vi "Set Travel Speed to Min or Max.vi"(8 "error in (no error)":errorcluster, 10 "Travel Speed":T1=enum."Minimum", 11 "ESM303 in":refnum<class "ESM303.lvclass">) -> (0 "error out":errorcluster, 3 "ESM303 out":refnum<class "ESM303.lvclass">)   [LabVIEW 2018, in "ESM303.lvlib" / "ESM303.lvclass"]
uses:
  ESM303.lvclass
  builds/Force Test Stand/Force Test Stand/Force Test Stand.lvlibp/Custom Controls/Travel Speed.ctl
  builds/Force Test Stand/Force Test Stand/Force Test Stand.lvlibp/Force Test Stand.lvclass
  C:/Projects/LabVIEW/In-Progress/Jose Rivero-Diaz/builds/Force Test Stand/Force Test Stand/Force Test Stand.lvlibp/Force Test Stand.lvclass
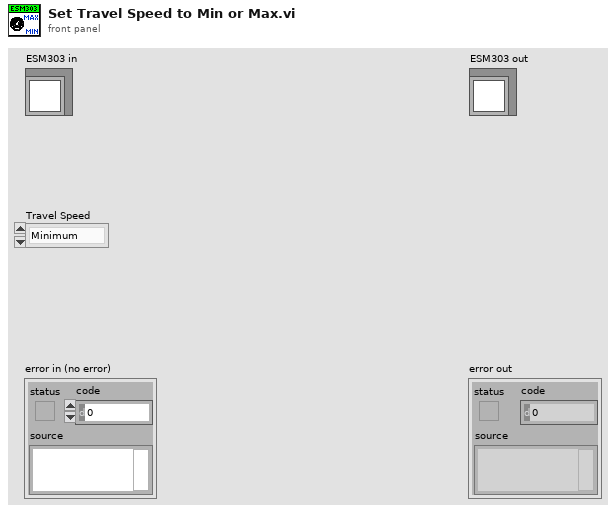
[diagram p1: front panel]
types:
  T1 = typedef "Force Test Stand.lvlibp/Force Test Stand.lvclass/Travel Speed.ctl" = enum16{"Maximum", "Minimum"}
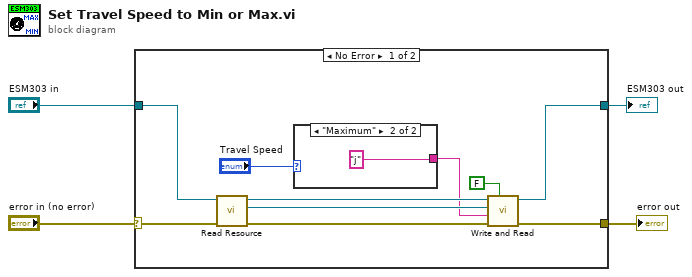
[diagram p0: block diagram]
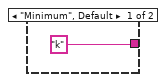
[diagram p2: hidden frame]
diagram:
  n1 = case shown="No Error" "error in (no error)" {
    selector: "error in (no error)" -> [w14 w18]
    tunnel: [w5 w18] -> w3
    tunnel: [w6 w17] -> w2
    tunnel: "ESM303 in" -> [w13 w17]
    frame No Error {
      n2 = call "Read Resource.vi"("error in (no error)"=w14, "Force Test Stand in"=w13) -> ("error out"=w12:errorcluster, "Resource"=w10:refnum<visa-resource-name>, "Force Test Stand out"=w11:refnum<class "ESM303.lvclass">)  [unwired: 7 in]
      n3 = case shown="\"Maximum\"" "Travel Speed" {
        tunnel: ["k" "j"] -> w8
        frame "Minimum", Default {
        }
        frame "Maximum" {
        }
      }
      n4 = call "Write and Read.vi"("Write & Read"=FALSE, "error in (no error)"=w12, "Command"=w8, "VISA Refnum in"=w10, "ESM303 in"=w11) -> ("error out"=w5:errorcluster, "ESM303 out"=w6:refnum<class "ESM303.lvclass">)  [unwired: 4 in, 1 out]
    }
    frame Error {
    }
  }
  "error out" <- w3
  "ESM303 out" <- w2
